vi "SWERVE_TRAJECTORY_EXECUTE.vi"(4 "Time Offset":dbl=-1.0 format="%16.4f", 6 "EnableClosedLoop":bool=TRUE, 8 "Init":bool, 9 "Reverse":bool, 10 "Follow Orientation":bool, 11 "Gyro Heading\nRAD":dbl) -> (0 "AtReference":bool, 1 "OutputTRAJ_STATE":T6={"TimeSeconds"=0.0, "Velocity"=0.0, "Acceleration"=0.0, "POSE"={"TRANSLATION"={"X"=0.0, "Y"=0.0}, "ROTATION"={"VALUE"=0.0, "COS"=1.0, "SIN"=0.0}}, "Curvature"=0.0} {"POSE"."ROTATION"."SIN" format="%13.4f"; "POSE"."ROTATION"."COS" format="%13.4f"; "POSE"."ROTATION"."VALUE" format="%13.4f"; "POSE"."TRANSLATION"."Y" format="%14.3f"; "POSE"."TRANSLATION"."X" format="%14.3f"}, 2 "Error and Corr":T4 {"Error Pose"."ROTATION"."SIN" format="%13.4f"; "Error Pose"."ROTATION"."COS" format="%13.4f"; "Error Pose"."ROTATION"."VALUE" format="%13.4f"; "Error Pose"."TRANSLATION"."Y" format="%14.3f"; "Error Pose"."TRANSLATION"."X" format="%14.3f"}, 3 "Chassis Velocity Target":T5 {"vOmega" format="%10.3f"; "vY" format="%10.3f"; "vX" format="%10.3f"}, 5 "Orientation Target":dbl)   [LabVIEW 2019]
uses:
  <vilib>/Rock Robotics/WPI/ThirdParty/JAS_Junk/TrajLib/TypeDef/TRAJ_STATE.ctl
  <vilib>/Rock Robotics/WPI/ThirdParty/JAS_Junk/TrajLib/TypeDef/POSE2D.ctl
  <vilib>/Rock Robotics/WPI/ThirdParty/JAS_Junk/TrajLib/TypeDef/TRANSLATION2D.ctl
  <vilib>/Rock Robotics/WPI/ThirdParty/JAS_Junk/TrajLib/TypeDef/ROTATION2D.ctl
  <vilib>/Rock Robotics/WPI/ThirdParty/JAS_Junk/TrajLib/TypeDef/CHASSIS_SPEEDS.ctl
  <vilib>/Rock Robotics/WPI/ThirdParty/JAS_Junk/TrajLib/ProfiledPIDController_NewPeriod.vi
  <vilib>/Rock Robotics/WPI/ThirdParty/JAS_Junk/TrajLib/ProfiledPIDController_SetIntegratorRange.vi
  <vilib>/Rock Robotics/WPI/ThirdParty/JAS_Junk/TrajLib/ProfiledPIDController_DisableContInput.vi
  <vilib>/Rock Robotics/WPI/ThirdParty/JAS_Junk/TrajLib/ProfiledPIDController_EnableContInput.vi
  <vilib>/Rock Robotics/WPI/ThirdParty/JAS_Junk/TrajLib/TrapProfConstraint_New.vi
  <vilib>/Rock Robotics/WPI/ThirdParty/JAS_Junk/TrajLib/VI/Util_GetTime_U32.vi
  <vilib>/Rock Robotics/WPI/ThirdParty/JAS_Junk/TrajLib/MathUtil_InputModulus.vi
  <vilib>/Rock Robotics/WPI/ThirdParty/JAS_Junk/TrajLib/HolDrvCtrl_New.vi
  <vilib>/Rock Robotics/WPI/ThirdParty/JAS_Junk/TrajLib/HolDrvCtrl_PackPID.vi
  <vilib>/Rock Robotics/WPI/ThirdParty/JAS_Junk/TrajLib/HolDrvCtrl_SetTolerance.vi
  <vilib>/Rock Robotics/WPI/ThirdParty/JAS_Junk/TrajLib/HolDrvCtrl_SetEnabled.vi
  <vilib>/Rock Robotics/WPI/ThirdParty/JAS_Junk/TrajLib/HolDrvCtrl_Calculate_Trajectory.vi
  <vilib>/Rock Robotics/WPI/ThirdParty/JAS_Junk/TrajLib/HolDrvCtrl_AtReference.vi
  <vilib>/Rock Robotics/WPI/ThirdParty/JAS_Junk/TrajLib/Rotation2d_UnaryMinus.vi
  <vilib>/Rock Robotics/WPI/ThirdParty/JAS_Junk/TrajLib/Rotation2d_RotateBy.vi
  <vilib>/Rock Robotics/WPI/ThirdParty/JAS_Junk/TrajLib/TrapProfState_New.vi
  <vilib>/Rock Robotics/WPI/ThirdParty/JAS_Junk/TrajLib/PIDController_NewPeriod.vi
  <vilib>/Rock Robotics/SystemInterfaces/NetworkCommunication/NetComm_UsageReport_report.vi
  <vilib>/Rock Robotics/WPI/ThirdParty/JAS_Junk/TrajLib/PIDController_SetIntegratorRange.vi
  <vilib>/Rock Robotics/WPI/ThirdParty/JAS_Junk/TrajLib/PIDController_DisableContinousInput.vi
  <vilib>/Rock Robotics/WPI/ThirdParty/JAS_Junk/TrajLib/PIDController_EnableContinousInput.vi
  <vilib>/Rock Robotics/WPI/ThirdParty/JAS_Junk/TrajLib/Conv_Deg_Radians.vi
  <vilib>/Rock Robotics/WPI/ThirdParty/JAS_Junk/TrajLib/PIDController_Reset.vi
  <vilib>/Rock Robotics/WPI/ThirdParty/JAS_Junk/TrajLib/HolDrvCtrl_Calculate.vi
  <vilib>/Rock Robotics/WPI/ThirdParty/JAS_Junk/TrajLib/Pose2d_getXYAngle.vi
  <vilib>/Rock Robotics/WPI/ThirdParty/JAS_Junk/TrajLib/Rotation2d_CreateXY.vi
  <vilib>/Rock Robotics/WPI/ThirdParty/JAS_Junk/TrajLib/Rotation2d_GetAngleCosSin.vi
  <vilib>/Rock Robotics/WPI/ThirdParty/JAS_Junk/TrajLib/Pose2d_RelativeTo.vi
  <vilib>/Rock Robotics/WPI/ThirdParty/JAS_Junk/TrajLib/ProfiledPIDController_Calculate_Meas_Goal.vi
  <vilib>/Rock Robotics/WPI/ThirdParty/JAS_Junk/TrajLib/ChassisSpeeds_FromFieldRelativeSpeeds.vi
  <vilib>/Rock Robotics/WPI/ThirdParty/JAS_Junk/TrajLib/PIDController_Calculate_SP_PV.vi
  <vilib>/Rock Robotics/WPI/ThirdParty/JAS_Junk/TrajLib/ProfiledPIDController_Reset_PosOnly.vi
  <vilib>/Rock Robotics/WPI/ThirdParty/JAS_Junk/TrajLib/Util_CalcDist.vi
  <vilib>/Rock Robotics/WPI/ThirdParty/JAS_Junk/TrajLib/Transform2d_Create_PosePose.vi
  <vilib>/Rock Robotics/WPI/ThirdParty/JAS_Junk/TrajLib/ProfiledPIDController_SetGoal_PosOnly.vi
  <vilib>/Rock Robotics/WPI/ThirdParty/JAS_Junk/TrajLib/ProfiledPIDController_Calculate_Meas.vi
  <vilib>/Rock Robotics/WPI/ThirdParty/JAS_Junk/TrajLib/Rotation2d_GetCos.vi
  <vilib>/Rock Robotics/WPI/ThirdParty/JAS_Junk/TrajLib/Rotation2d_GetSin.vi
  <vilib>/Rock Robotics/WPI/ThirdParty/JAS_Junk/TrajLib/PIDController_SetSetpoint.vi
  <vilib>/Rock Robotics/WPI/ThirdParty/JAS_Junk/TrajLib/PIDController_Calculate_PV.vi
  <vilib>/Rock Robotics/WPI/ThirdParty/JAS_Junk/TrajLib/ProfiledPIDController_Reset.vi
  <vilib>/Rock Robotics/WPI/ThirdParty/JAS_Junk/TrajLib/Translation2d_RotateBy.vi
  <vilib>/Rock Robotics/WPI/ThirdParty/JAS_Junk/TrajLib/Translation2d_Minus.vi
  <vilib>/Rock Robotics/WPI/ThirdParty/JAS_Junk/TrajLib/ProfiledPIDController_SetGoal.vi
  <vilib>/Rock Robotics/WPI/ThirdParty/JAS_Junk/TrajLib/TrapProfile_New.vi
  <vilib>/Rock Robotics/WPI/ThirdParty/JAS_Junk/TrajLib/ProfiledPIDController_GetPeriod.vi
  <vilib>/Rock Robotics/WPI/ThirdParty/JAS_Junk/TrajLib/TrapProfile_Calculate.vi
  <vilib>/Rock Robotics/WPI/ThirdParty/JAS_Junk/TrajLib/ControllerUtil_GetModulusError.vi
  <vilib>/Rock Robotics/WPI/ThirdParty/JAS_Junk/TrajLib/Translation2d_Create.vi
  <vilib>/Rock Robotics/WPI/ThirdParty/JAS_Junk/TrajLib/TrapProfile_ShouldFlipAcceleration.vi
  <vilib>/Rock Robotics/WPI/ThirdParty/JAS_Junk/TrajLib/TrapProfile_Direct.vi
  <vilib>/Rock Robotics/WPI/ThirdParty/JAS_Junk/TrajLib/PIDController_GetPeriod.vi
  Swerve_Drive_System/SWERVE_DRIVE_GLOBALS.vi
  <vilib>/Rock Robotics/WPI/ThirdParty/JAS_Junk/TrajLib/Globals/Util_LibraryGlobals.vi
  <vilib>/Rock Robotics/WPI/ThirdParty/JAS_Junk/TrajLib/VI/Util_GetTime_U64.vi
  <vilib>/Rock Robotics/WPI/ThirdParty/JAS_Junk/TrajLib/Trajectory_Library.lvlib
panel:
  # "(FOR TESTING)"
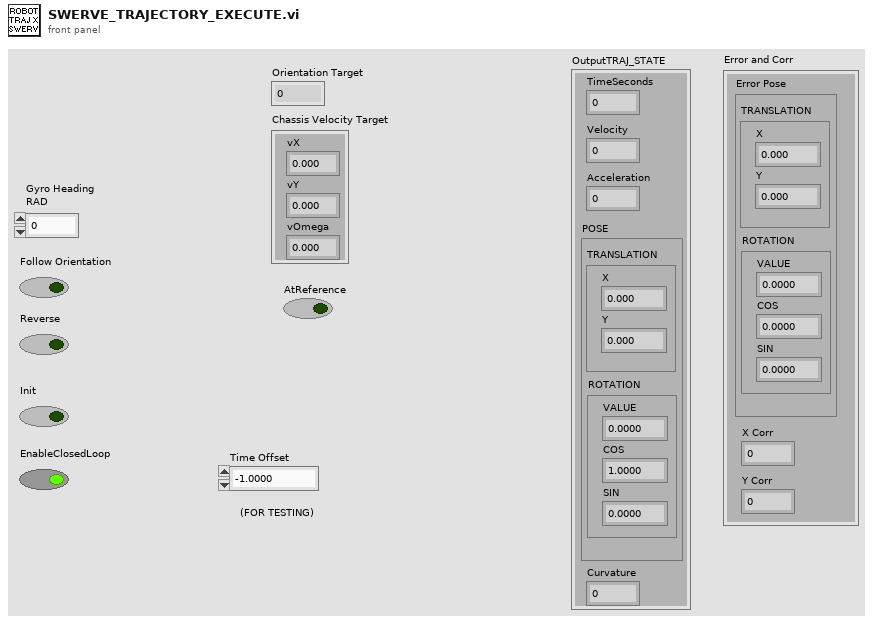
[diagram p1: front panel]
types:
  T1 = typedef "Trajectory_Library.lvlib/POSE2D.ctl" = cluster{"TRANSLATION":T2, "ROTATION":T3}
  T2 = typedef "Trajectory_Library.lvlib/TRANSLATION2D.ctl" = cluster{"X":dbl, "Y":dbl}
  T3 = typedef "Trajectory_Library.lvlib/ROTATION2D.ctl" = cluster{"VALUE":dbl, "COS":dbl, "SIN":dbl}
  T4 = cluster{"Error Pose":T1, "X Corr":dbl, "Y Corr":dbl}
  T5 = typedef "Trajectory_Library.lvlib/CHASSIS_SPEEDS.ctl" = cluster{"vX":dbl, "vY":dbl, "vOmega":dbl}
  T6 = typedef "Trajectory_Library.lvlib/TRAJ_STATE.ctl" = cluster{"TimeSeconds":dbl, "Velocity":dbl, "Acceleration":dbl, "POSE":T1, "Curvature":dbl}
  T7 = typedef "Trajectory_Library.lvlib/SWERVE_DRIVE_KINEMATICS.ctl" = cluster{"NumModules":i32, "InverseKinematics":T8, "ForwardKinematics":T8, "Modules":T2[], "PrevCoR":T2, "SavedModuleStates":T9[]}
  T8 = typedef "NI_Matrix.lvlib/RealMatrix.ctl" = dbl[][]
  T9 = typedef "Trajectory_Library.lvlib/SWERVE_DRIVE_MODULE_STATE.ctl" = cluster{"Speed":dbl, "Angle":T3}
  T10 = typedef "Trajectory_Library.lvlib/SWERVE_DRIVE_MODULE_POSITION.ctl" = cluster{"Distance":dbl, "Angle":T3, "P":bool}
  T11 = typedef "Trajectory_Library.lvlib/TRAJECTORY.ctl" = cluster{"TotalTImeSecs":dbl, "States":T6[]}
  T12 = typedef "Trajectory_Library.lvlib/PID_TUNING.ctl" = cluster{"Kp":dbl, "Ki":dbl, "Kd":dbl, "MaximumIntegral":dbl, "MinimumIntegral":dbl}
  T13 = typedef "Trajectory_Library.lvlib/PROFILED_PID_CONTROLLER.ctl" = cluster{"Controller":T14, "Goal":T15, "Setpoint":T15, "Constraint":T16}
  T14 = typedef "Trajectory_Library.lvlib/PID_CONTROLLER.ctl" = cluster{"Kp":dbl, "Ki":dbl, "Kd":dbl, "Period":dbl, "Max_Integral":dbl, "Min_Integral":dbl, "Max_Input":dbl, "Min_Input":dbl, "Continuous":bool, "PositionError":dbl, "VelocityError":dbl, "PrevError":dbl, "TotalError":dbl, "PositionTolerance":dbl, "VelocityTolerance":dbl, "SetPoint":dbl, "Kf":dbl, "Prev_Deriv":dbl, "Prev_Deriv 2":dbl, "DerivativeFilter":bool, "Min_Output":dbl, "Max_Output":dbl, "Prev_F_P":dbl, "Prev_F_P_2":dbl, "AntiWindupActive":bool, "Measurement":dbl}
  T15 = typedef "Trajectory_Library.lvlib/TRAPEZOID_PROFILE_STATE.ctl" = cluster{"Position":dbl, "Velocity":dbl}
  T16 = typedef "Trajectory_Library.lvlib/TRAPEZOID_PROFILE_CONSTRAINT.ctl" = cluster{"MaxVelocity":dbl, "MaxAcceleration":dbl}
  T17 = typedef "Trajectory_Library.lvlib/HOLONOMIC_DRV_CTRL.ctl" = cluster{"poseTolerance":T1, "poseError":T1, "Enabled":bool, "PID_xCtrl":T14, "PID_yCtrl":T14, "PROF_PID_thetaCtrl":T13, "RotationError":T3, "FirstRun":bool}
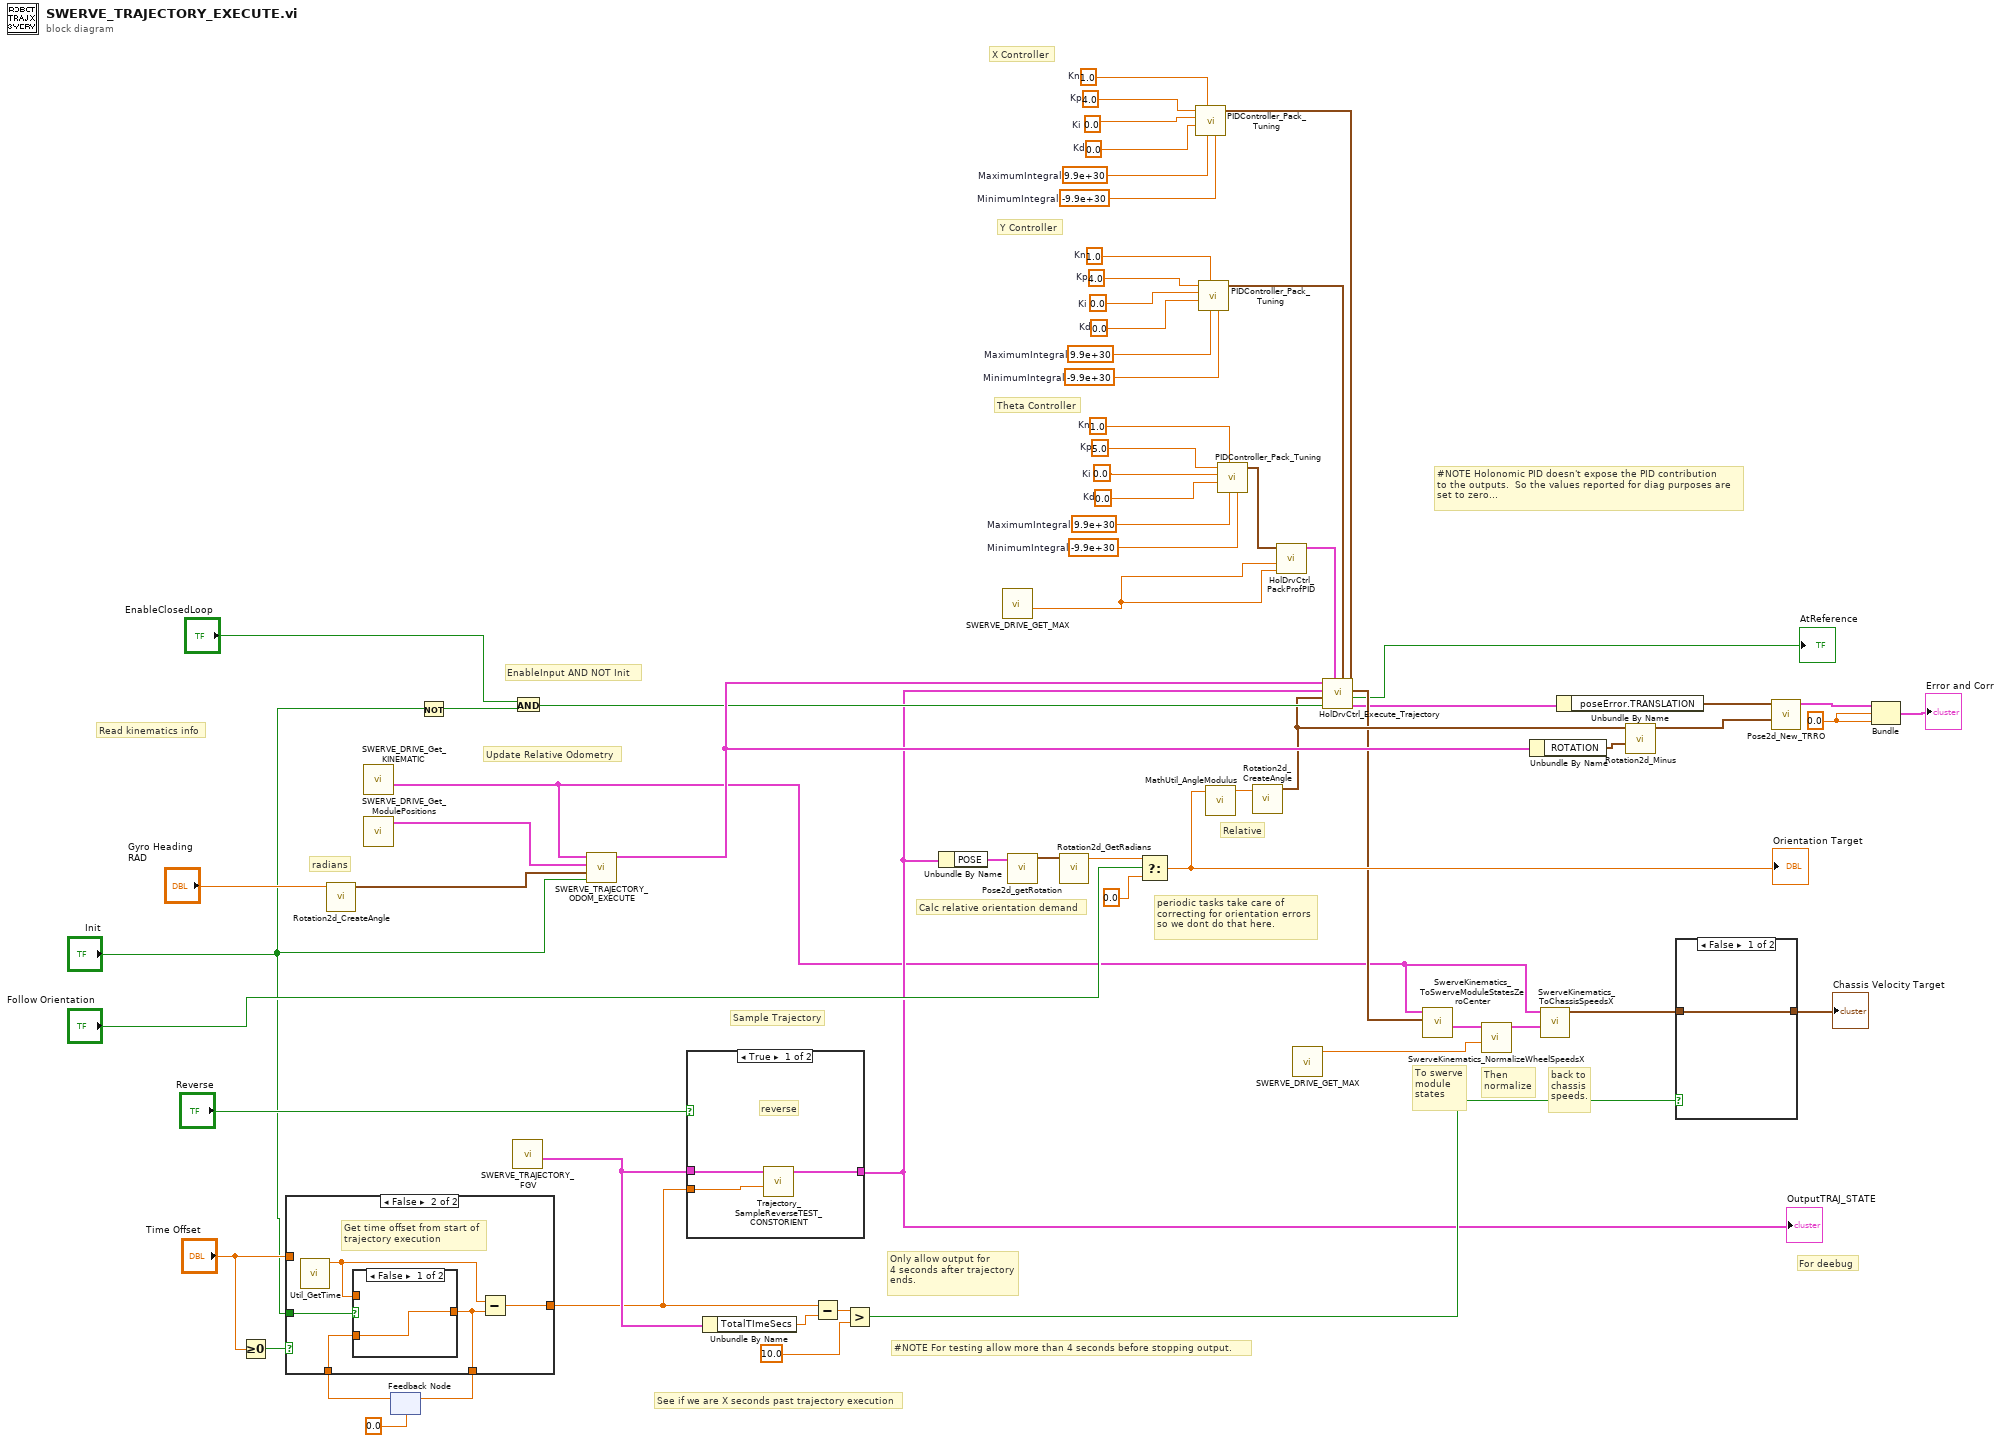
[diagram p0: block diagram]
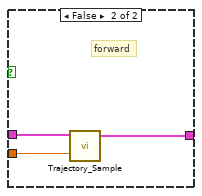
[diagram p4: hidden frame]
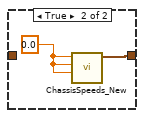
[diagram p5: hidden frame]
diagram:
  w20 = 1.0  # Kn
  w23 = 5.0  # Kp
  w32 = 0.0  # Ki
  w33 = 0.0  # Kd
  w34 = 9.9e+30  # MaximumIntegral
  w35 = -9.9e+30  # MinimumIntegral
  w18 = 1.0  # Kn
  w21 = 4.0  # Kp
  w24 = 0.0  # Ki
  w25 = 0.0  # Kd
  w26 = 9.9e+30  # MaximumIntegral
  w27 = -9.9e+30  # MinimumIntegral
  w19 = 1.0  # Kn
  w22 = 4.0  # Kp
  w28 = 0.0  # Ki
  w29 = 0.0  # Kd
  w30 = 9.9e+30  # MaximumIntegral
  w31 = -9.9e+30  # MinimumIntegral
  w46 = 0.0
  # "For deebug"
  # "Update Relative Odometry"
  # "#NOTE For testing allow more than 4 seconds before stopping output."
  # "EnableInput AND NOT Init"
  # "Theta Controller"
  # "Y Controller"
  # "X Controller"
  # "Relative"
  # "#NOTE Holonomic PID doesn't expose the PID contribution \nto the outputs.  So the values reported for diag purposes are\nset to zero..."
  # "back to\nchassis\nspeeds."
  # "Then\nnormalize"
  # "To swerve\nmodule\nstates"
  # "Calc relative orientation demand"
  # "Read kinematics info"
  # "Sample Trajectory"
  # "See if we are X seconds past trajectory execution"
  # "radians"
  # "periodic tasks take care of\ncorrecting for orientation errors\nso we dont do that here."
  # "Only allow output for\n4 seconds after trajectory\nends."
  n1 = Greater Or Equal To 0?(x="Time Offset") -> (x >= 0?=w50:bool)
  n2 = call <vilib>:"Rotation2d_CreateAngle.vi"("Angle"="Gyro Heading\nRAD") -> ("ROTATION"=w6:T3)  [unwired: 10 in]
  n3 = call "SWERVE_DRIVE_Get_KINEMATIC.vi"() -> ("out SWERVE_DRIVE_KINEMATICS"=w4:T7)  [unwired: 11 in]
  n4 = call "SWERVE_DRIVE_Get_ModulePositions.vi"() -> ("Swerve Module Positions"=w3:T10[])  [unwired: 11 in]
  n5 = feedback #1(0.0 ("TIME")) -> (w52:dbl)
  n6 = case shown="False" w50 {
    tunnel: [w68 w74] -> w65
    tunnel: "Init" -> [_ w72]
    tunnel: w52 -> [w69 w71]
    tunnel: [w69 w70] -> w51
    tunnel: "Time Offset" -> [w68 _]
    frame True {
      # "For testing allow\nuser entered time offset!!"
    }
    frame False {
      # "Get time offset from start of\ntrajectory execution"
      n7 = call <vilib>:"Util_GetTime.vi"() -> ("FPGA_Time_Seconds"=w73:dbl)  [unwired: 9 in, 2 out]
      n8 = case shown="False" w72 {
        tunnel: [w75 w76] -> w70
        tunnel: w71 -> [w75 _]
        tunnel: w73 -> [_ w76]
        frame False {
        }
        frame True {
        }
      }
      n9 = Subtract(x=w73, y=w70) -> (x-y=w74:dbl)
    }
  }
  n10 = feedback-in #1(w51) -> ()
  n11 = Not(x="Init") -> (.not. x?=w47:bool)
  n12 = call "SWERVE_TRAJECTORY_FGV.vi"() -> ("outTRAJECTORY"=w67:T11)  [unwired: 11 in]
  n13 = And(x="EnableClosedLoop", y=w47) -> (x .and. y?=w11:bool)
  n14 = call "SWERVE_TRAJECTORY_ODOM_EXECUTE.vi"("Init"="Init", "ROTATION"=w6, "Swerve Module Positions"=w3, "out SWERVE_DRIVE_KINEMATICS"=w4) -> ("robot POSE"=w12:T1)  [unwired: 5 in, 2 out]
  n15 = case shown="True" "Reverse" {
    tunnel: w67 -> [w79 w82]
    tunnel: w65 -> [w77 w81]
    tunnel: [w78 w80] -> w10
    frame True {
      # "reverse"
      n16 = call "Trajectory_SampleReverseTEST_CONSTORIENT.vi"("Time"=w77, "InputTRAJECTORY"=w79) -> ("OutputTRAJ_STATE"=w78:T6)  [unwired: 9 in]
    }
    frame False {
      # "forward"
      n17 = call <vilib>:"Trajectory_Sample.vi"("Time"=w81, "InputTRAJECTORY"=w82) -> ("OutputTRAJ_STATE"=w80:T6)  [unwired: 9 in]
    }
  }
  "OutputTRAJ_STATE" <- w10
  n18 = Unbundle By Name(w67) -> ("TotalTImeSecs"=w66:dbl)
  n19 = Subtract(x=w65, y=w66) -> (x-y=w64:dbl)
  n20 = Greater?(x=w64, y=10.0) -> (0:w62:bool)
  n21 = Unbundle By Name(w10) -> ("POSE"=w54:T1)
  n22 = call "SWERVE_DRIVE_GET_MAX.vi"() -> ("Max Rotational Vel (Rad/Sec)"=w13:dbl)  [unwired: 10 in, 1 out]
  n23 = call <vilib>:"Pose2d_getRotation.vi"("in POSE"=w54) -> ("out ROTATION"=w58:T3)  [unwired: 10 in]
  n24 = call <vilib>:"Rotation2d_GetRadians.vi"("in ROTATION"=w58) -> ("AngleRadians"=w39:dbl)  [unwired: 10 in]
  n25 = Select(t=w39, s="Follow Orientation", f=0.0) -> (s? t:f=w36:dbl)
  "Orientation Target" <- w36
  n26 = call <vilib>:"PIDController_Pack_Tuning.vi"("MinimumIntegral"=w27, "MaximumIntegral"=w26, "Kn"=w18, "Kd"=w25, "Ki"=w24, "Kp"=w21) -> ("PID Tuning"=w14:T12)  [unwired: 5 in]
  n27 = call <vilib>:"PIDController_Pack_Tuning.vi"("MinimumIntegral"=w31, "MaximumIntegral"=w30, "Kn"=w19, "Kd"=w29, "Ki"=w28, "Kp"=w22) -> ("PID Tuning"=w15:T12)  [unwired: 5 in]
  n28 = call <vilib>:"MathUtil_AngleModulus.vi"("InputAngle"=w36) -> ("ModulsAngle"=w45:dbl)  [unwired: 10 in]
  n29 = call <vilib>:"PIDController_Pack_Tuning.vi"("MinimumIntegral"=w35, "MaximumIntegral"=w34, "Kn"=w20, "Kd"=w33, "Ki"=w32, "Kp"=w23) -> ("PID Tuning"=w17:T12)  [unwired: 5 in]
  n30 = call <vilib>:"Rotation2d_CreateAngle.vi"("Angle"=w45) -> ("ROTATION"=w9:T3)  [unwired: 10 in]
  n31 = call <vilib>:"HolDrvCtrl_PackProfPID.vi"("Max Accel"=w13, "Max Speed"=w13, "Theta PID Tuning"=w17) -> ("Theta PID CONTROLLER"=w16:T13)  [unwired: 8 in]
  n32 = call "SWERVE_DRIVE_GET_MAX.vi"() -> ("Max Wheel Vel (Meter/Sec)"=w55:dbl)  [unwired: 10 in, 1 out]
  n33 = call <vilib>:"HolDrvCtrl_Execute_Trajectory.vi"("X PID Tuning"=w14, "Y PID Tuning"=w15, "thetaProfiledPID_CTRL"=w16, "Enable"=w11, "angleRef"=w9, "desiredTrajState"=w10, "currentPose"=w12) -> ("outHOLONOMIC_DRV_CTRL"=w7:T17, "AtReference"=→"AtReference":bool, "calcChassisSpeed"=w8:T5)  [unwired: 2 in]
  n34 = call <vilib>:"SwerveKinematics_ToSwerveModuleStatesZeroCenter.vi"("ChassisSpeeds"=w8, "in SWERVE_DRIVE_KINEMATICS"=w4) -> ("ModuleStates"=w60:T9[])  [unwired: 8 in, 1 out]
  n35 = call <vilib>:"SwerveKinematics_NormalizeWheelSpeedsX.vi"("AttainableMaxSpeed"=w55, "in WheelStates"=w60) -> ("out WheelStates"=w59:T9[])  [unwired: 9 in]
  n36 = Unbundle By Name(w12) -> ("ROTATION"=w40:T3)
  n37 = call <vilib>:"SwerveKinematics_ToChassisSpeedsX.vi"("WheelStates"=w59, "in SWERVE_DRIVE_KINEMATICS"=w4) -> ("Chassis Speed"=w5:T5)  [unwired: 9 in]
  n38 = Unbundle By Name(w7) -> ("poseError.TRANSLATION"=w44:T2)
  n39 = call <vilib>:"Rotation2d_Minus.vi"("other ROTATION"=w40, "in ROTATION"=w9) -> ("out ROTATION"=w43:T3)  [unwired: 9 in]
  n40 = case shown="False" w62 {
    tunnel: w5 -> [w83 _]
    tunnel: [w83 w84] -> w56
    frame False {
    }
    frame True {
      w85 = 0.0 ("vX")
      n41 = call <vilib>:"ChassisSpeeds_New.vi"("vAngular"=w85, "vY"=w85, "vX"=w85) -> ("CHASSIS"=w84:T5)  [unwired: 8 in]
    }
  }
  "Chassis Velocity Target" <- w56
  n42 = call <vilib>:"Pose2d_New_TRRO.vi"("ROTATION"=w43, "TRANSLATION"=w44) -> ("outPOSE"=w42:T1)  [unwired: 9 in]
  n43 = Bundle("outPOSE"=w42, w46, w46) -> (→"Error and Corr":cluster{"outPOSE":T1, dbl, dbl})  [unwired: 1 in]
